vi "AI Data Cluster Conversion.vi"(8 "error in":errorcluster, 9 "1D array?":bool, 10 "Waveform Cluster":T2(array[cluster]), 11 "Input 1D Cluster":T4(array[cluster])) -> (0 "error out":errorcluster, 2 "Waveform Array":T1(array[cluster]), 3 "1D Array":T3(array[cluster]))   [LabVIEW 2024]
doc: "All Rights Reserved © 2017 SyncSols"
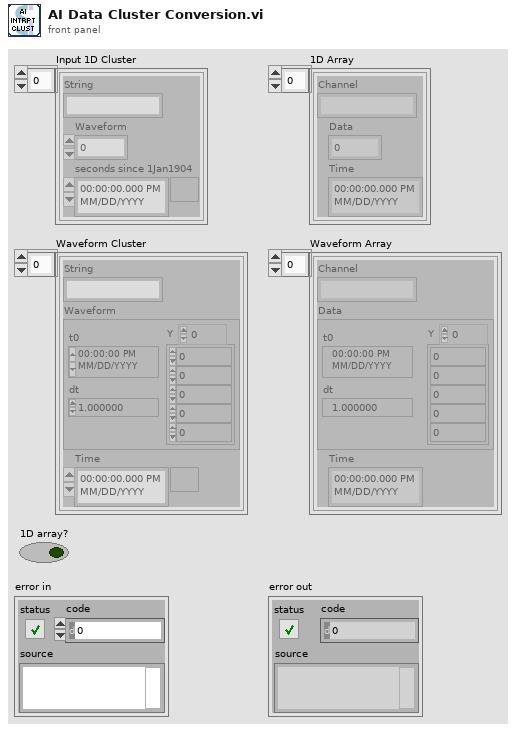
[diagram p1: front panel]
types:
  T1 = cluster{"Channel":string, "Data":waveform(dbl), "Time":timestamp}[]
  T2 = cluster{"String":string, "Waveform":waveform(dbl), "Time":timestamp}[]
  T3 = cluster{"Channel":string, "Data":dbl, "Time":timestamp}[]
  T4 = cluster{"String":string, "Waveform":dbl, "seconds since 1Jan1904":timestamp}[]
  T5 = cluster{"Channel":string, "Data":dbl, "Time":timestamp}
  T6 = cluster{"Channel":string, "Data":waveform(dbl), "Time":timestamp}
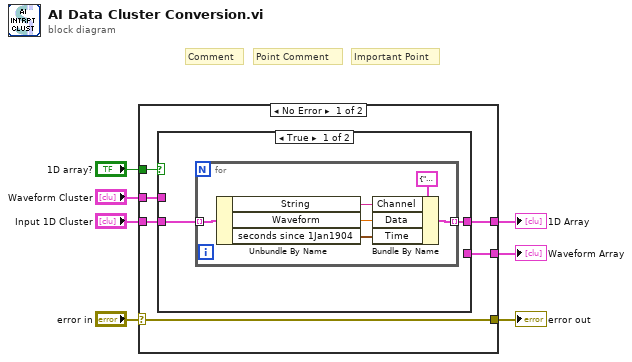
[diagram p0: block diagram]
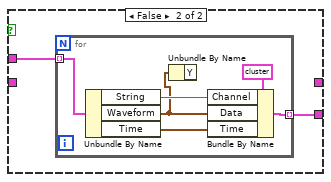
[diagram p2: hidden frame]
diagram:
  # "Important Point"
  # "Point Comment"
  # "Comment"
  n1 = case shown="No Error" "error in" {
    selector: "error in" -> [w13 w30]
    tunnel: [w13 w30] -> w7
    tunnel: "Input 1D Cluster" -> [w12 _]
    tunnel: [w11 _] -> w4
    tunnel: "1D array?" -> [w10 _]
    tunnel: "Waveform Cluster" -> [w9 _]
    tunnel: [w8 _] -> w1
    frame No Error {
      n2 = case shown="True" w10 {
        tunnel: w12 -> [w15 _]
        tunnel: [w14 _] -> w11
        tunnel: w9 -> [_ w23]
        tunnel: [_ w22] -> w8
        frame True {
          n3 = for {
            tunnel: w15 -> [w21] mode=indexing
            tunnel: [w17] -> w14 mode=indexing
            n4 = Unbundle By Name(w21) -> ("String"=w20:string, "Waveform"=w19:dbl, "seconds since 1Jan1904"=w18:timestamp)
            n5 = Bundle By Name(cluster=T5 {"Channel"="", "Data"=0.0, "Time"=timestamp(0 s since 1904-01-01)} ("Cluster"), "Channel"=w20, "Data"=w19, "Time"=w18) -> (w17:T5)
          }
        }
        frame False {
          n6 = for {
            tunnel: w23 -> [w29] mode=indexing
            tunnel: [w27] -> w22 mode=indexing
            n7 = Unbundle By Name(w29) -> ("String"=w28:string, "Waveform"=w24:waveform(dbl), "Time"=w26:timestamp)
            n8 = Unbundle By Name(w24) -> ()  [unwired: 1 out]
            n9 = Bundle By Name(cluster=T6 {"Channel"="", "Data"={"t0"=timestamp(0 s since 1904-01-01), "dt"=1.0, "Y"=[]}, "Time"=timestamp(0 s since 1904-01-01)} ("Cluster"), "Channel"=w28, "Data"=w24, "Time"=w26) -> (w27:T6)
          }
        }
      }
    }
    frame Error {
    }
  }
  "error out" <- w7
  "1D Array" <- w4
  "Waveform Array" <- w1
